vi "End.vi"(8 "error in (no error)":errorcluster, 11 "Experiment3D in":refnum<class "Experiment3D.lvclass">) -> (0 "error out":errorcluster, 3 "Experiment3D out":refnum<class "Experiment3D.lvclass">)   [LabVIEW 2014, in "Experiment3D.lvclass"]
uses:
  Experiment3D.lvclass
  Measurement/Measurement3D/Measurement3D.lvclass
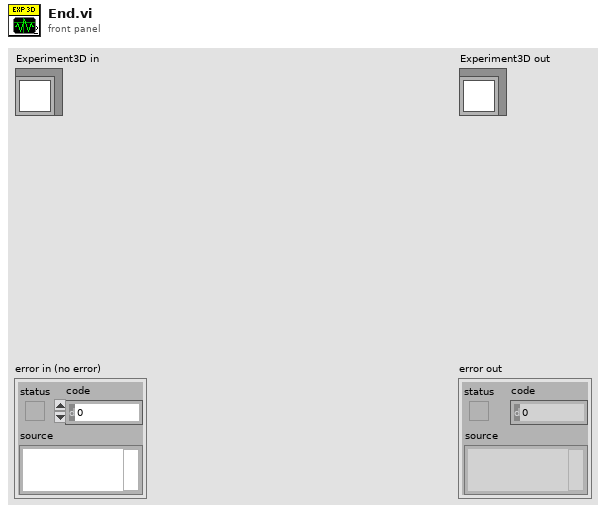
[diagram p1: front panel]
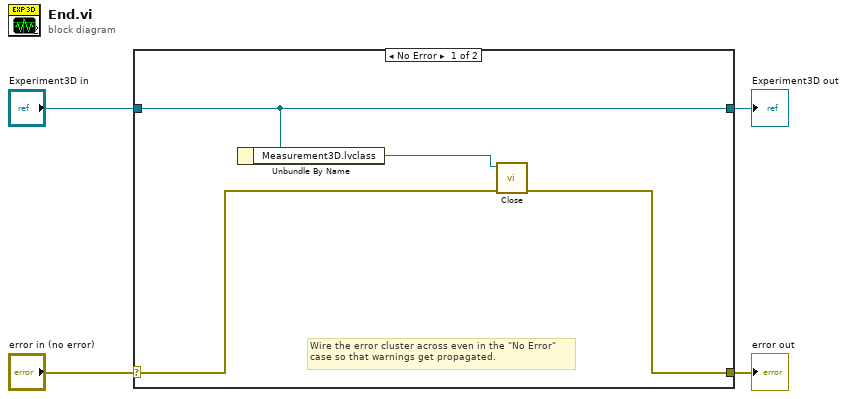
[diagram p0: block diagram]
diagram:
  n1 = case shown="No Error" "error in (no error)" {
    selector: "error in (no error)" -> [w6 w10]
    tunnel: [w5 w10] -> w3
    tunnel: [w8 w9] -> w1
    tunnel: "Experiment3D in" -> [w8 w9]
    frame No Error {
      # "Wire the error cluster across even in the \"No Error\"\ncase so that warnings get propagated."
      n2 = Unbundle By Name(w8) -> ("Measurement3D.lvclass"=w7:refnum<class "Measurement3D.lvclass">)
      n3 = call "Close.vi"("error in (no error)"=w6, "Measurement3D in"=w7) -> ("error out"=w5:errorcluster)  [unwired: 8 in, 1 out]
    }
    frame Error {
    }
  }
  "error out" <- w3
  "Experiment3D out" <- w1
